vi "Compile - Rx Channel Refs.vi"(7 "Packet Name":string, 8 "error in (no error)":errorcluster, 11 "Item Ref in":T1 format="%.0x") -> (0 "error out":errorcluster, 3 "Item Ref out":T1 format="%.0x", 5 "Rx Ref Array":T2(array[cluster]) {"VS Refs" format="%.0x"})   [LabVIEW 2019, in "UDP-Custom-Device System Explorer.lvlib"]
uses:
  UDP-Custom-Device System Explorer.lvlib
  <vilib>/NI VeriStand/Custom Device API/Custom Device Item Ref.ctl
  <vilib>/NI VeriStand/Custom Device Tools/Custom Device Utility Library/Custom Device Utility Library.lvlib
  <vilib>/NI VeriStand/Custom Device API/Custom Device API.lvlib
  Property Accessors/Rx Channel Section Accessors.lvlib
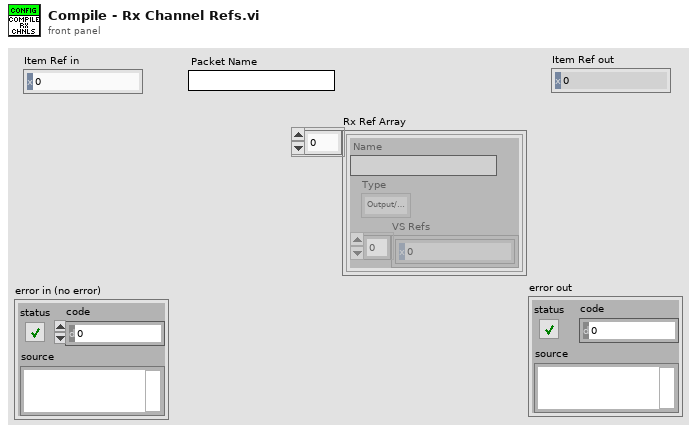
[diagram p1: front panel]
types:
  T1 = typedef "Custom Device API.lvlib/Custom Device Item Ref.ctl" = u64
  T2 = cluster{"Name":string, "Type":enum16{"Output/Write", "Input/Read", "Input/ReadWrite"}, "VS Refs":T1[]}[]
  T3 = enum16{"Output/Write", "Input/Read", "Input/ReadWrite"}
  T4 = cluster{"Name":string, "Type":enum16{"Output/Write", "Input/Read", "Input/ReadWrite"}, "VS Refs":T1[]}
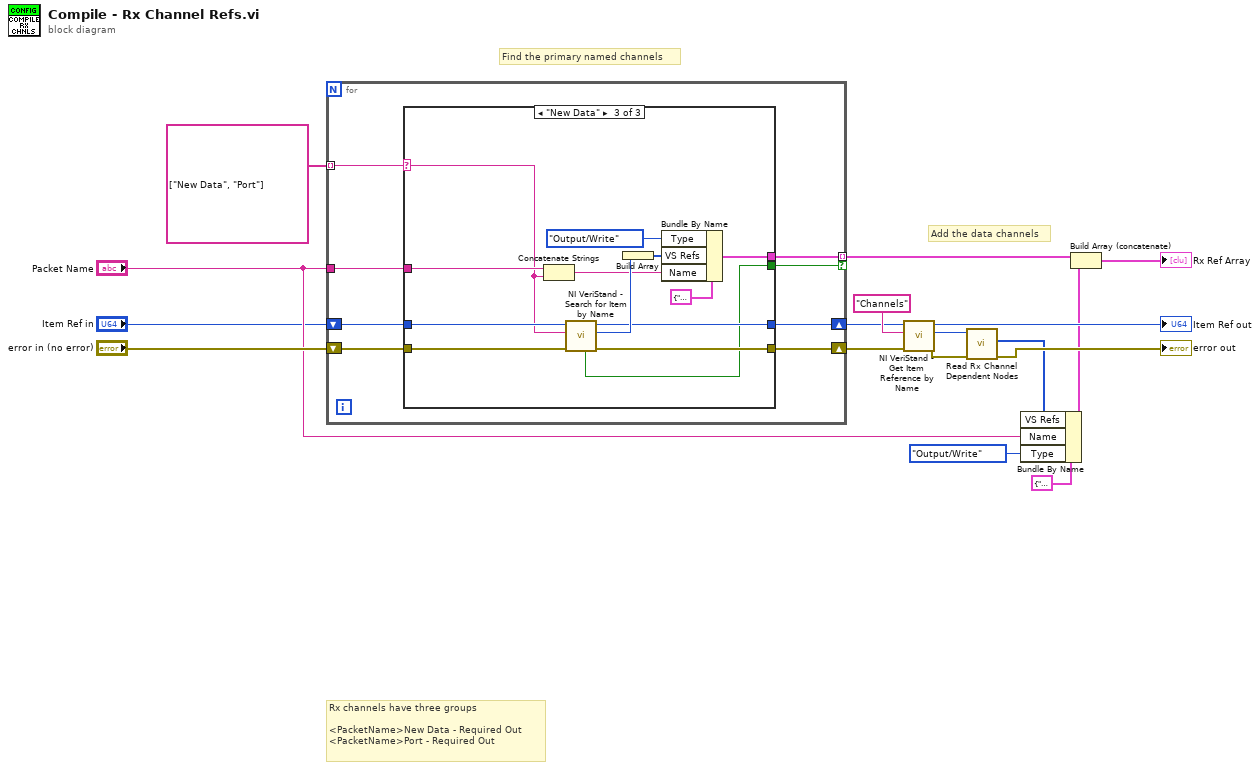
[diagram p0: block diagram]
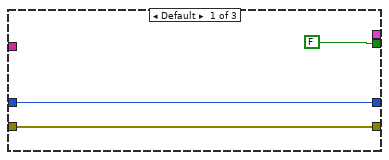
[diagram p2: hidden frame]
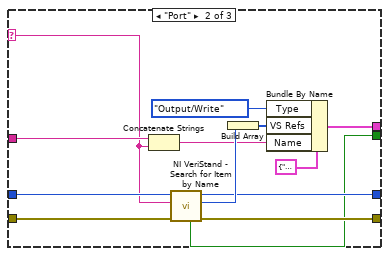
[diagram p3: hidden frame]
diagram:
  # "Add the data channels"
  # "Find the primary named channels"
  # "Rx channels have three groups\n\n<PacketName>New Data - Required Out\n<PacketName>Port - Required Out"
  n1 = for {
    tunnel: string[] ["New Data", "Port"] ("Item GUID") -> [w25] mode=indexing
    tunnel: "Packet Name" -> [w20]
    tunnel: [w22] -> w4 mode=indexing if=w21
    shift-right: [w19] -> w6
    shift-left: "Item Ref in" -> [w23]
    shift-right: [w18] -> w5
    shift-left: "error in (no error)" -> [w24]
    n2 = case shown="\"New Data\"" w25 {
      selector: w25 -> [_ w30 w43]
      tunnel: w24 -> [w27 w36 w49]
      tunnel: w23 -> [w28 w37 w50]
      tunnel: [w28 w35 w48] -> w19
      tunnel: [w27 w34 w47] -> w18
      tunnel: [_ w33 w46] -> w22
      tunnel: [FALSE ("Found") w32 w45] -> w21
      tunnel: w20 -> [_ w31 w44]
      frame Default {
      }
      frame "Port" {
        n3 = Concatenate Strings(w31, w30) -> (w29:string)
        n4 = call <vilib>:"NI VeriStand - Search for Item by Name.vi"("error in"=w36, "Item Name"=w30, "Section Ref in"=w37) -> ("error out"=w34:errorcluster, "Item Ref"=w39:T1, "Section Ref out"=w35:T1, "Found"=w32:bool)  [unwired: 5 in]
        n5 = Build Array(w39) -> (w40:T1[])
        n6 = Bundle By Name(cluster=T4 {"Name"="", "Type"=enum."Output/Write", "VS Refs"=[]} ("Group"), "Type"=T3."Output/Write", "VS Refs"=w40, "Name"=w29) -> (w33:T4)
      }
      frame "New Data" {
        n7 = Concatenate Strings(w44, w43) -> (w42:string)
        n8 = call <vilib>:"NI VeriStand - Search for Item by Name.vi"("error in"=w49, "Item Name"=w43, "Section Ref in"=w50) -> ("error out"=w47:errorcluster, "Item Ref"=w52:T1, "Section Ref out"=w48:T1, "Found"=w45:bool)  [unwired: 5 in]
        n9 = Build Array(w52) -> (w53:T1[])
        n10 = Bundle By Name(cluster=T4 {"Name"="", "Type"=enum."Output/Write", "VS Refs"=[]} ("Group"), "Type"=T3."Output/Write", "VS Refs"=w53, "Name"=w42) -> (w46:T4)
      }
    }
  }
  n11 = call <vilib>:"NI VeriStand - Get Item Reference by Name.vi"("error in (no error)"=w5, "Item Name"="Channels" ("Section Name"), "Parent Ref in"=w6) -> ("error out"=w8:errorcluster, "Item Ref"=w9:T1, "Parent Ref out"=→"Item Ref out":T1)  [unwired: 5 in, 1 out]
  n12 = call "Read Rx Channel Dependent Nodes.vi"("error in (no error)"=w8, "Node Ptr"=w9) -> ("error out"=→"error out":errorcluster, "Dependent Node Refs"=w2:T1[])  [unwired: 7 in, 1 out]
  n13 = Bundle By Name(cluster=T4 {"Name"="", "Type"=enum."Output/Write", "VS Refs"=[]} ("Group"), "VS Refs"=w2, "Name"="Packet Name", "Type"=T3."Output/Write") -> (w3:T4)
  n14 = Build Array (concatenate)(w4, w3) -> (→"Rx Ref Array":T2)
